vi "Connect.vi"(8 "error in (no error)":errorcluster, 11 "6512 in":refnum<class "6512.lvclass">) -> (0 "error out":errorcluster, 3 "6512 out":refnum<class "6512.lvclass">)   [LabVIEW 2019, in "6512.lvlib" / "6512.lvclass"]
uses:
  Library/6512.lvclass
  C:/Users/Public/Documents/Development/builds/Instruments/Instruments.lvlibp/Library/Instruments.lvclass
  Library/6512.lvclass/6512.ctl
  builds/Instruments/Instruments.lvlibp/Accessors/Read Resource.vi
  <resource>/objmgr/daqmx.rc
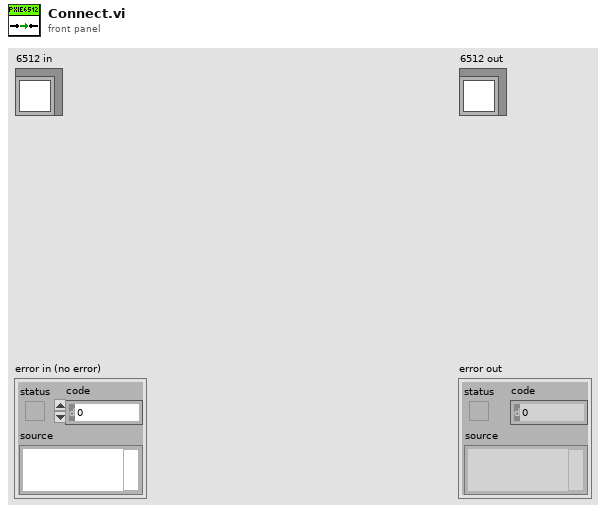
[diagram p1: front panel]
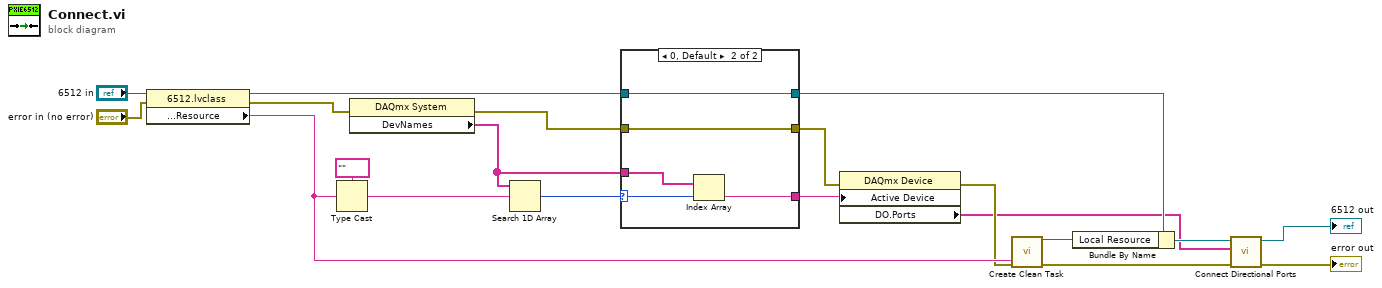
[diagram p0: block diagram]
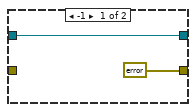
[diagram p2: hidden frame]
diagram:
  n1 = property class="6512.lvclass"(reference="6512 in", error in="error in (no error)") -> (reference out=w7:refnum<class "6512.lvclass">, error out=w16:errorcluster, "Accessors:Configuration:Resource"=w17:string)
  n2 = Type Cast(type=tag "" ("DAQmx Device Name"), x=w17) -> (*(type *) &x=w12:tag)
  n3 = property class="DAQmx System"(error in=w16) -> (error out=w10:errorcluster, "DevNames"=w14:tag[])  [unwired: 1 in, 1 out]
  n4 = Search 1D Array(1D array=w14, element=w12) -> (index of element=w5:i32)  [unwired: 1 in]
  n5 = case shown="0, Default" w5 {
    selector: w5 -> [_ w23]
    tunnel: w14 -> [_ w27]
    tunnel: [_ w26] -> w11
    tunnel: w10 -> [_ w25]
    tunnel: [errorcluster {"status"=TRUE, "code"=1, "source"="Device not found"} ("error out") w25] -> w9
    tunnel: w7 -> [w21 w24]
    tunnel: [w21 w24] -> w6
    frame -1 {
    }
    frame 0, Default {
      n6 = Index Array(array=w27, index=w23) -> (element=w26:tag)
    }
  }
  n7 = property class="DAQmx Device"(error in=w9, "Active Device"=w11) -> (error out=w8:errorcluster, "DO.Ports"=w1:tag[])  [unwired: 1 in, 1 out]
  n8 = call "Create Clean Task.vi"("Task Name"=w17, "error in (no error)"=w8) -> ("error out"=w4:errorcluster, "task out"=w2:refnum<k21>)  [unwired: 8 in]
  n9 = Bundle By Name(cluster=w6, "Local Resource"=w2) -> (w3:refnum<class "6512.lvclass">)
  n10 = call "Connect Directional Ports.vi"("error in"=w4, "Digital Ports"=w1, "6512 in"=w3) -> ("error out"=→"error out":errorcluster, "6512 out"=→"6512 out":refnum<class "6512.lvclass">)  [unwired: 7 in]
